vi "Get_FV_Para_MC_List.vi"(7 "View":bool, 8 "error in (no error)":errorcluster, 10 "Machine No.":string, 11 "Refnum in":T1) -> (0 "error out":errorcluster, 1 "Search Queary":string, 2 "Column":string[](array[string]), 3 "Refnum out":T1, 4 "Column Display":string[](array[string]), 5 "Table":string)   [LabVIEW 2020]
uses:
  <vilib>/addons/database/Connection.llb/Conn ObjectReference.ctl
  <userlib>/_OpenG.lib/array/array.llb/Search 1D Array (Boolean)__ogtk.vi
  <userlib>/_OpenG.lib/array/array.llb/Delete Elements from 1D Array (String)__ogtk.vi
  <vilib>/addons/database/_DB Variant To Data/Database Variant To Data.xnode
  <vilib>/addons/database/NI_Database_API.lvlib
panel:
  out "resulting string":string
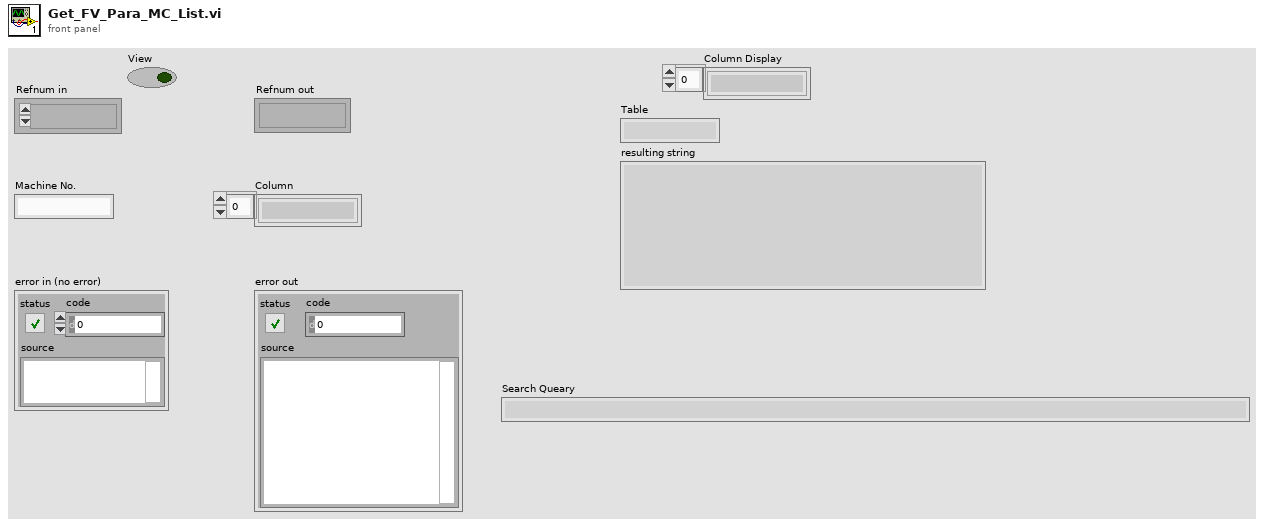
[diagram p1: front panel]
types:
  T1 = typedef "NI_Database_API.lvlib/Conn ObjectReference.ctl" = refnum<k1>
  T2 = typedef "TD SQL.ctl" = cluster{"MS SQL Connection":T1, "UDL File":path, "Time":string, "DCODE":string, "WIP+1":i64, "MC No?":i32, "POKAYOKE?":bool, "Expected Result":string, "Result [Status]":string, "Clock":dbl, "RFID":string, "WIP Queue":refnum<queue>, "TS Parameter":T3, "Data_Queue":refnum<queue>[], "RFID Serial No.":string}
  T3 = typedef "TS_Parameter.ctl" = cluster{"ProfitCenterCode":string, "LineCode":string, "WorkOrderNumber":string, "Model":string, "Model_with_Prefix":string, "VendorCode":string, "SetParameterDateCode":string, "PokaYoke":i32, "Target":i32, "Live_DateCode":string, "CustomerPartNumber":string, "Hand":string, "Ent_Stamp":timestamp, "STS_CD":dbl}
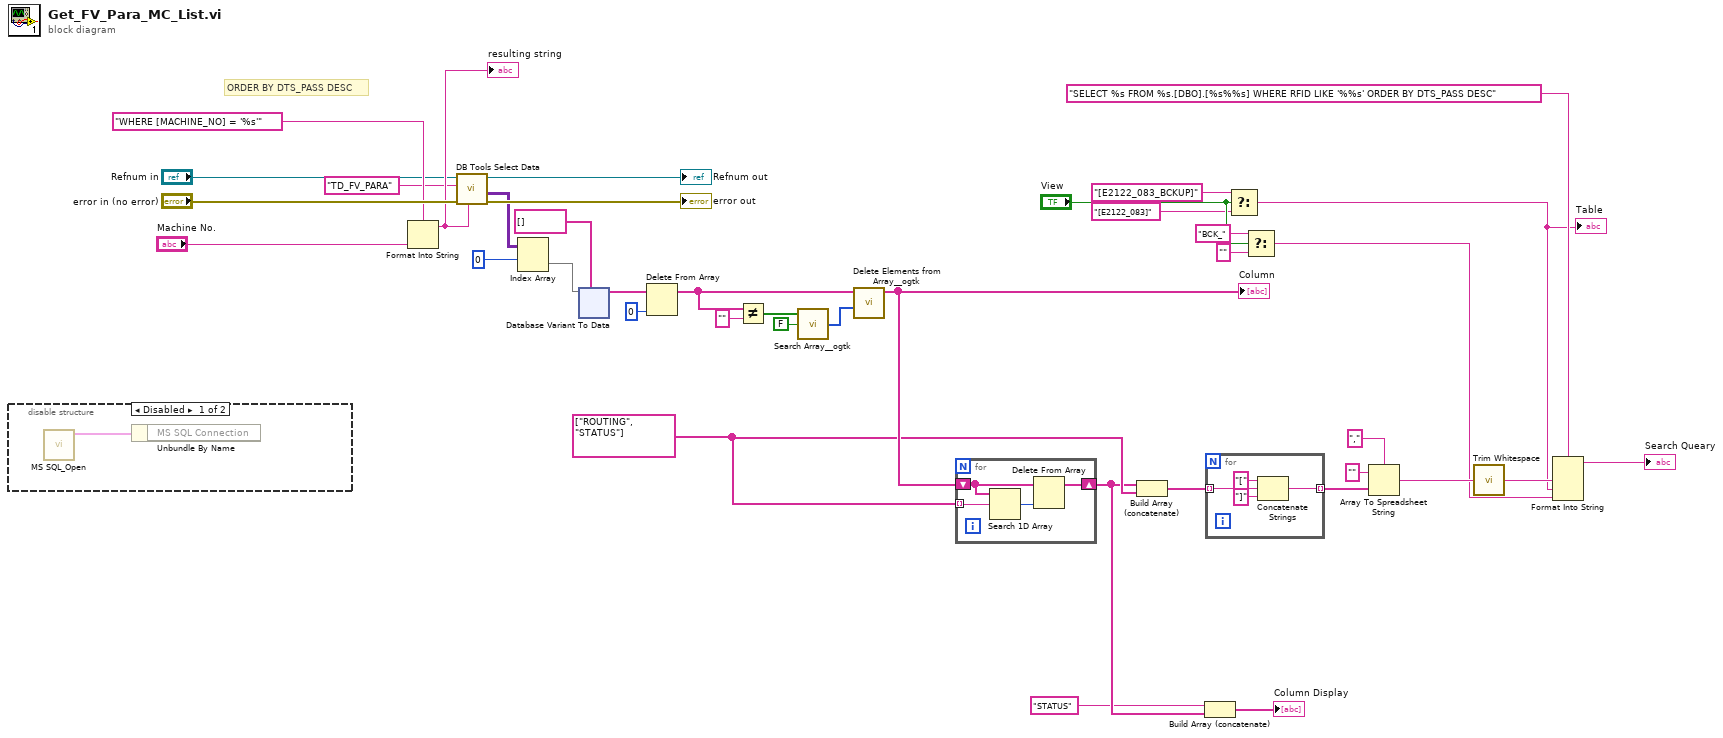
[diagram p0: block diagram]
diagram:
  w20 = string[] ["ROUTING", "STATUS"] ("array w/ subset deleted")
  # "ORDER BY DTS_PASS DESC"
  n1 = disable-structure shown="Disabled" {
    frame Disabled {
      n2 = call "MS SQL_Open.vi"() -> ("Ref Out"=w41:T2)  [unwired: 9 in, 2 out]
      n3 = Unbundle By Name(w41) -> ("MS SQL Connection"=w40:T1)
    }
    frame Enabled {
    }
  }
  n4 = Format Into String(format string="WHERE [MACHINE_NO] = '%s'" ("condition"), "Machine No.") -> (resulting string=w24:string)  [unwired: 2 in, 1 out]
  "resulting string" <- w24
  n5 = call <vilib>:"DB Tools Select Data.vi"("condition"=w24, "error in (no error)"="error in (no error)", "table"="TD_FV_PARA", "connection reference"="Refnum in") -> ("error out"=→"error out":errorcluster, "data"=w25:variant[][], "connection reference out"=→"Refnum out":T1)  [unwired: 2 in]
  n6 = Index Array(array=w25, index (row)=0) -> (element=w27:variant[])  [unwired: 1 in]
  n7 = xnode "Database Variant To Data"("database variant"=w27, "type"=string[] [] ("columns")) -> ("data"=w29:string[])  [unwired: 1 in, 1 out]
  n8 = Delete From Array(array=w29, index=0) -> (array with subset deleted=w38:string[])  [unwired: 1 in, 1 out]
  n9 = Not Equal?(x=w38, y="" ("resulting string")) -> (x != y?=w35:bool[])
  n10 = call-poly <userlib>:"Search Array__ogtk.vi"("Array"=w35, "Element Data"=FALSE) -> ("Indices of Elements"=w37:i32[])  [unwired: 7 in]
  n11 = call-poly <userlib>:"Delete Elements from Array__ogtk.vi"("indices"=w37, "array"=w38) -> ("array w/ subset deleted"=w21:string[])  [unwired: 8 in, 1 out]
  "Column" <- w21
  n12 = for {
    shift-right: [w42] -> w11
    shift-left: w21 -> [w44]
    tunnel: w20 -> [w45] mode=indexing
    n13 = Search 1D Array(1D array=w44, element=w45) -> (index of element=w43:i32)  [unwired: 1 in]
    n14 = Delete From Array(array=w44, index=w43) -> (array with subset deleted=w42:string[])  [unwired: 1 in, 1 out]
  }
  n15 = Build Array (concatenate)(w11, w20) -> (w19:string[])
  n16 = Build Array (concatenate)("STATUS", w11) -> (→"Column Display":string[])
  n17 = for {
    tunnel: w19 -> [w49] mode=indexing
    tunnel: [w46] -> w18 mode=indexing
    n18 = Concatenate Strings("[" ("string"), w49, "]" ("string")) -> (w46:string)
  }
  n19 = Select(t="[E2122_083_BCKUP]" ("format string"), s="View", f="[E2122_083]" ("format string")) -> (s? t:f=w3:string)
  "Table" <- w3
  n20 = Select(t="BCK_", s="View", f="") -> (s? t:f=w2:string)
  n21 = Array To Spreadsheet String(delimiter (Tab)=",", array=w18, 3:"" ("format string")) -> (spreadsheet string=w14:string)
  n22 = call <vilib>:"Trim Whitespace.vi"("string"=w14) -> ("trimmed string"=w12:string)  [unwired: 1 in]
  n23 = Format Into String(format string="SELECT %s FROM %s.[DBO].[%s%%s] WHERE RFID LIKE '%%s' ORDER BY DTS_PASS DESC" ("String"), w12, w3, w2) -> (resulting string=→"Search Queary":string)  [unwired: 2 in, 1 out]
